vi "Set Timing Source.vi"(8 "error in":errorcluster, 10 "hardware parameters":T1, 11 "module handle":u32) -> (0 "error out":errorcluster, 3 "module handle out":u32)   [LabVIEW 2020, in "AIM MIL-STD-1553 Hardware API.lvlib"]
uses:
  AIM MIL-STD-1553 Hardware API.lvlib
  Shared/AIM Hardware Parameters.ctl
  Shared/Initialization Method.ctl
  Shared/Bus Selection.ctl
  Shared/Coupling Mode.ctl
  Shared/Timing Mode.ctl
  <instrlib>/_AIM MIL-STD-1553/PCI-1553 Mid-Level Release/1553 Utility - RT Mode Global.vi
  Global - Disable Hardware API Constant.vi
  <vilib>/NI VeriStand/Custom Device Tools/Custom Device Utility Library/Custom Device Utility Library.lvlib
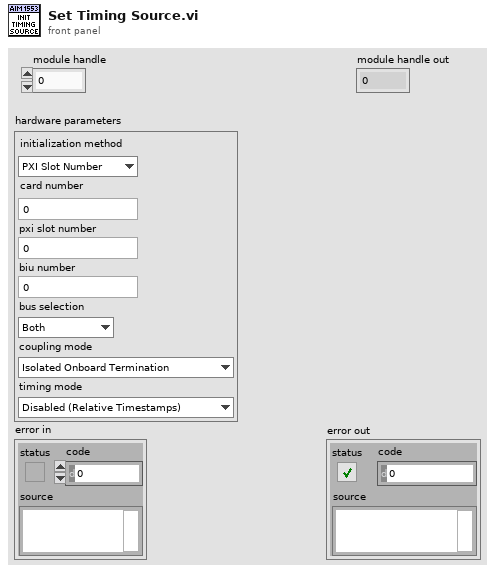
[diagram p1: front panel]
types:
  T1 = typedef "AIM Hardware Parameters.ctl" = cluster{"initialization method":T2, "card number":i32, "pxi slot number":i32, "biu number":i32, "bus selection":T3, "coupling mode":T4, "timing mode":T5}
  T2 = typedef "Initialization Method.ctl" = enum16{"PXI Slot Number", "Card Number"}
  T3 = typedef "Bus Selection.ctl" = enum16{"Both", "Primary", "Secondary"}
  T4 = typedef "Coupling Mode.ctl" = enum16{"Isolated Onboard Termination", "Transformer Coupled", "Direct Coupled", "External with Onboard Termination", "Onboard Digital Wrap-around"}
  T5 = typedef "Timing Mode.ctl" = enum16{"Disabled (Relative Timestamps)", "IRIG (Internal System Time)", "IRIG (External Timing Source)"}
  T6 = enum16{"Enabled (Default)", "Disabled for Unit Testing"}
  T7 = cluster{"Days of year":u32, "Hours":u32, "Minutes":u32, "Seconds":u32, "Milliseconds":u32}
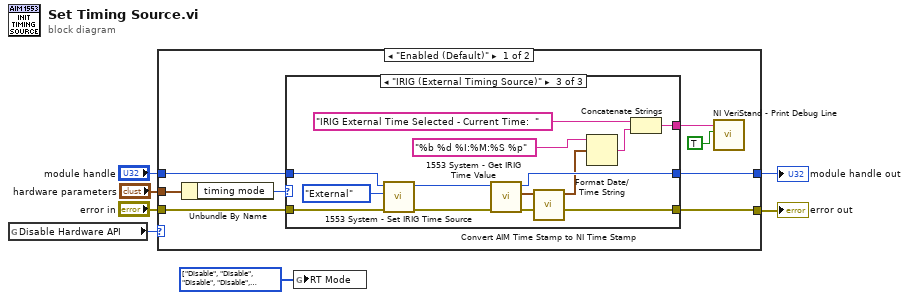
[diagram p0: block diagram]
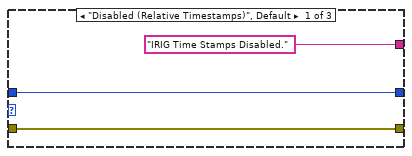
[diagram p2: hidden frame]
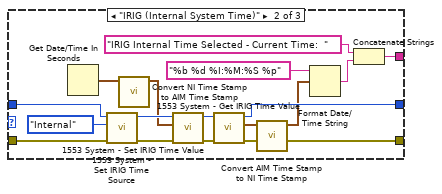
[diagram p3: hidden frame]
diagram:
  w2 = enum16{"Disable", "Simulation", "Monitor"}[] [enum."Disable", enum."Disable", enum."Disable", enum."Disable", enum."Disable", enum."Disable", enum."Disable", enum."Disable", enum."Disable", enum."Disable", enum."Disable", enum."Disable", enum."Disable", enum."Disable", enum."Disable", enum."Disable", enum."Disable", enum."Disable", enum."Disable", enum."Disable", enum."Disable", enum."Disable", enum."Disable", enum."Disable", enum."Disable", enum."Disable", enum."Disable", enum."Disable", enum."Disable", enum."Disable", enum."Disable", enum."Disable"] items=["Disable", "Simulation", "Monitor"] ("RT Mode")
  n1 = global read "Global - Disable Hardware API Constant.vi" "Disable Hardware API"() -> (w3:T6)
  n2 = case shown="\"Enabled (Default)\"" w3 {
    tunnel: [w13 w50] -> w7
    tunnel: "error in" -> [w14 w50]
    tunnel: [w11 w49] -> w5
    tunnel: "hardware parameters" -> [w15 _]
    tunnel: "module handle" -> [w12 w49]
    frame "Enabled (Default)" {
      n3 = Unbundle By Name(w15) -> ("timing mode"=w10:T5)
      n4 = case shown="\"IRIG (External Timing Source)\"" w10 {
        tunnel: w14 -> [w17 w35 w48]
        tunnel: [w17 w32 w43] -> w13
        tunnel: w12 -> [w18 w34 w47]
        tunnel: [w18 w31 w42] -> w11
        tunnel: ["IRIG Time Stamps Disabled." w27 w37] -> w8
        frame "Disabled (Relative Timestamps)", Default {
        }
        frame "IRIG (Internal System Time)" {
          n5 = Get Date/Time In Seconds() -> (seconds since 1Jan1904=w19:timestamp)
          n6 = call <instrlib>:"1553 System - Set IRIG Time Source.vi"("Error In (none)"=w35, "Time Source (internal)"=enum16{"Internal", "External"}."Internal", "Module Handle"=w34) -> ("Error Out"=w25:errorcluster, "Module Handle Output"=w24:u32)  [unwired: 7 in]
          n7 = call "Convert NI Time Stamp to AIM Time Stamp.vi"("Time Stamp"=w19) -> ("IRIG Time Stamp"=w21:T7)  [unwired: 10 in]
          n8 = call <instrlib>:"1553 System - Set IRIG Time Value.vi"("Error In (none)"=w25, "IRIG Time Stamp"=w21, "Module Handle"=w24) -> ("Error Out"=w22:errorcluster, "Module Handle Output"=w23:u32)  [unwired: 7 in]
          n9 = call <instrlib>:"1553 System - Get IRIG Time Value.vi"("Error In (none)"=w22, "Module Handle"=w23) -> ("Error Out"=w32:errorcluster, "IRIG Time Stamp"=w20:T7, "Module Handle Output"=w31:u32)  [unwired: 7 in]
          n10 = call "Convert AIM Time Stamp to NI Time Stamp.vi"("IRIG Time Stamp"=w20) -> ("Time Stamp"=w30:timestamp)  [unwired: 10 in]
          n11 = Format Date/Time String(time format string (%c)="%b %d %I:%M:%S %p", seconds (now)=w30) -> (date/time string=w29:string)  [unwired: 1 in]
          n12 = Concatenate Strings("IRIG Internal Time Selected - Current Time:  ", w29) -> (w27:string)
        }
        frame "IRIG (External Timing Source)" {
          n13 = call <instrlib>:"1553 System - Set IRIG Time Source.vi"("Error In (none)"=w48, "Time Source (internal)"=enum16{"Internal", "External"}."External", "Module Handle"=w47) -> ("Error Out"=w44:errorcluster, "Module Handle Output"=w45:u32)  [unwired: 7 in]
          n14 = call <instrlib>:"1553 System - Get IRIG Time Value.vi"("Error In (none)"=w44, "Module Handle"=w45) -> ("Error Out"=w43:errorcluster, "IRIG Time Stamp"=w41:T7, "Module Handle Output"=w42:u32)  [unwired: 7 in]
          n15 = call "Convert AIM Time Stamp to NI Time Stamp.vi"("IRIG Time Stamp"=w41) -> ("Time Stamp"=w40:timestamp)  [unwired: 10 in]
          n16 = Format Date/Time String(time format string (%c)="%b %d %I:%M:%S %p", seconds (now)=w40) -> (date/time string=w39:string)  [unwired: 1 in]
          n17 = Concatenate Strings("IRIG External Time Selected - Current Time:  ", w39) -> (w37:string)
        }
      }
      n18 = call <vilib>:"NI VeriStand - Print Debug Line.vi"("Add to log file? (F)"=TRUE, "Message"=w8) -> ()  [unwired: 9 in, 1 out]
    }
    frame "Disabled for Unit Testing" {
    }
  }
  "error out" <- w7
  "module handle out" <- w5
  n19 = global write "1553 Utility - RT Mode Global.vi" "RT Mode"(w2) -> ()
